vi "SweepCtrlStepCal_DP_ver1.0.vi"(0 "Run Cluster":T1 {"Main Sweep" items=["Time", "DC Current", "Delta Current", "Pulse Delta Current", "Sine Current", "Lock-in Vosc"]; "Magnet Control (IPS 120-10)"."Action" items=["Hold", "To Set point", "To Zero", "Clamp"]; "Keithley 6221 :"."Sweep Mode" items=["Linear", "Log", "Exp", "Inverse", "Manual"]}) -> (1 "Stay duration pts":dbl[](array[numeric]), 2 "2D Array of DC Source or Lock-In Ctrl Run Cluster":cluster{"GPIB ADR":u16, "DC St. Pt.":dbl}[][](array[cluster]))   [LabVIEW 2011]
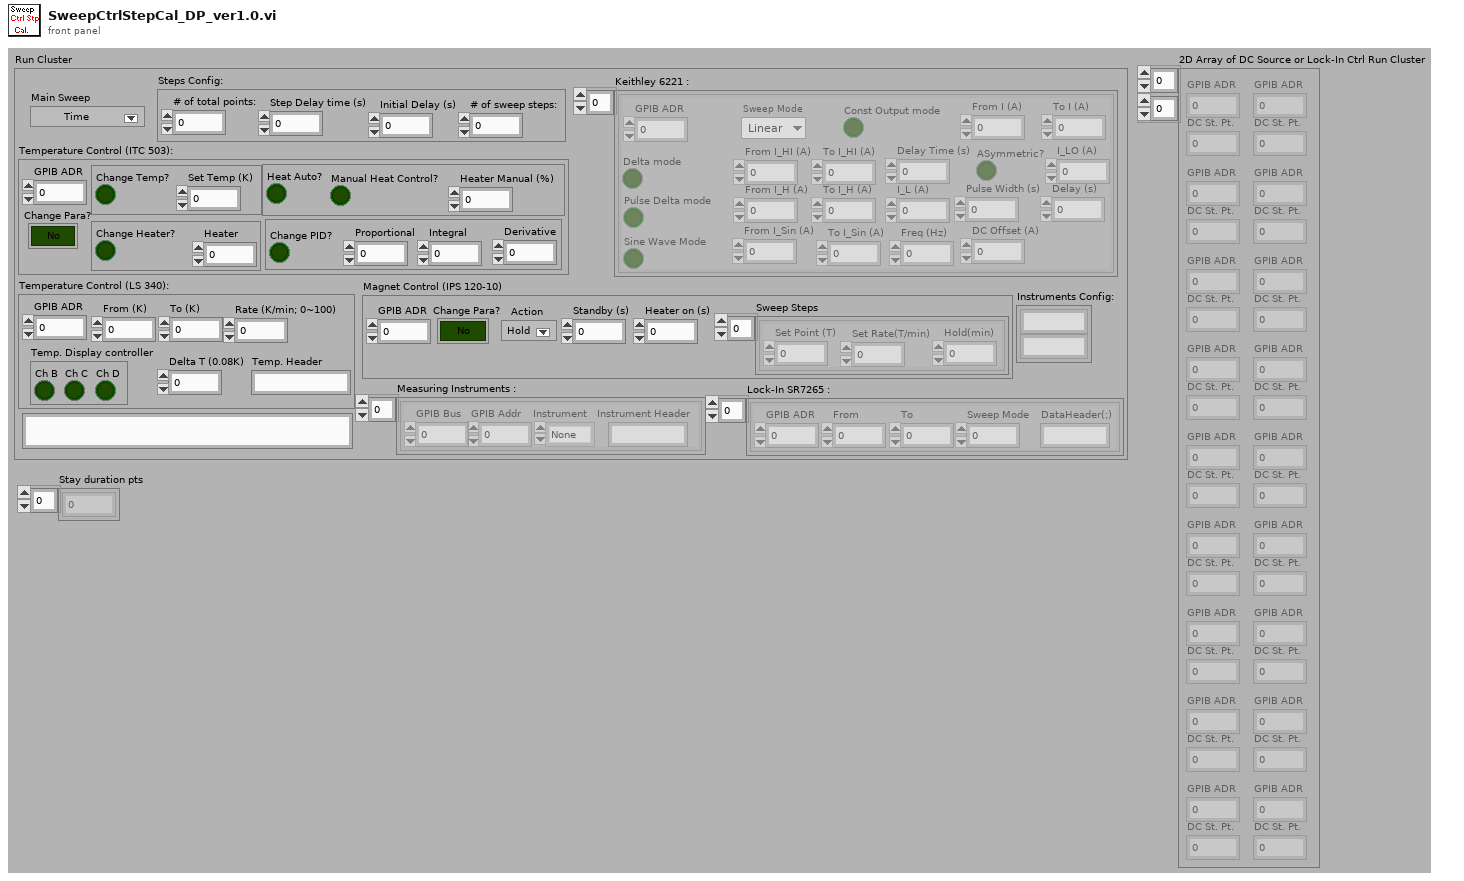
[diagram p1: front panel]
types:
  T1 = cluster{"Main Sweep":u8, "Steps Config:":cluster{"# of total points:":u32, "Step Delay time (s)":dbl, "Initial Delay (s)":dbl, "# of sweep steps:":u32}, "Temperature Control (ITC 503):":cluster{"GPIB ADR":u16, "Change Heater?":cluster{"Change Heater?":bool, "Heater":u8}, "Change Temp?":cluster{"Change Temp?":bool, "Set Temp (K)":dbl}, "Cluster":cluster{"Heat Auto?":bool, "Manual Heat Control?":bool, "Heater Manual (%)":dbl}, "Change PID?":cluster{"Change PID?":bool, "Proportional":dbl, "Integral":dbl, "Derivative":dbl}, "Change Para?":bool}, "Temperature Control (LS 340):":cluster{"GPIB ADR":u16, "From (K)":dbl, "To (K)":dbl, "Rate (K/min; 0~100)":dbl, "Delta T (0.08K)":dbl, "Temp. Header":string, "Temp. Display controller":cluster{"Ch B":bool, "Ch C":bool, "Ch D":bool}}, "Magnet Control (IPS 120-10)":cluster{"Action":u16, "Standby (s)":dbl, "Heater on (s)":dbl, "Sweep Steps ":cluster{"Set Point (T)":dbl, "Set Rate(T/min)":dbl, "Hold(min)":dbl}[], "GPIB ADR":u16, "Change Para?":bool}, "Keithley 6221 :":cluster{"Delta mode":bool, "Const Output mode":bool, "Pulse Delta mode":bool, "Sine Wave Mode":bool, "From I_HI (A)":dbl, "From I (A)":dbl, "I_LO (A)":dbl, "From I_H (A)":dbl, "I_L (A)":dbl, "Freq (Hz)":dbl, "From I_Sin (A)":dbl, "DC Offset (A)":dbl, "Delay Time (s)":dbl, "Pulse Width (s)":dbl, "Delay (s)":dbl, "To I (A)":dbl, "ASymmetric?":bool, "To I_HI (A)":dbl, "To I_H (A)":dbl, "To I_Sin (A)":dbl, "GPIB ADR":u16, "Sweep Mode":u8}[], "Measuring Instruments : ":cluster{"GPIB Bus":dbl, "GPIB Addr":dbl, "Instrument":enum16{"None", "HP34401DMM", "Lockin 7265", "HP3456/7A", "HP3478A", "HP3325FG"}, "Instrument Header":string}[], "Lock-In SR7265 :":cluster{"GPIB ADR":u16, "From":dbl, "To":dbl, "DataHeader(;)":string, "Sweep Mode":u8}[], "Deascription of \nthis measurement":string, "Instruments Config:":string[][]}
  T2 = cluster{"# of total points:":u32, "Step Delay time (s)":dbl, "Initial Delay (s)":dbl, "# of sweep steps:":u32}
  T3 = cluster{"GPIB ADR":u16, "From":dbl, "To":dbl, "DataHeader(;)":string, "Sweep Mode":u8}[]
  T4 = cluster{"Delta mode":bool, "Const Output mode":bool, "Pulse Delta mode":bool, "Sine Wave Mode":bool, "From I_HI (A)":dbl, "From I (A)":dbl, "I_LO (A)":dbl, "From I_H (A)":dbl, "I_L (A)":dbl, "Freq (Hz)":dbl, "From I_Sin (A)":dbl, "DC Offset (A)":dbl, "Delay Time (s)":dbl, "Pulse Width (s)":dbl, "Delay (s)":dbl, "To I (A)":dbl, "ASymmetric?":bool, "To I_HI (A)":dbl, "To I_H (A)":dbl, "To I_Sin (A)":dbl, "GPIB ADR":u16, "Sweep Mode":u8}[]
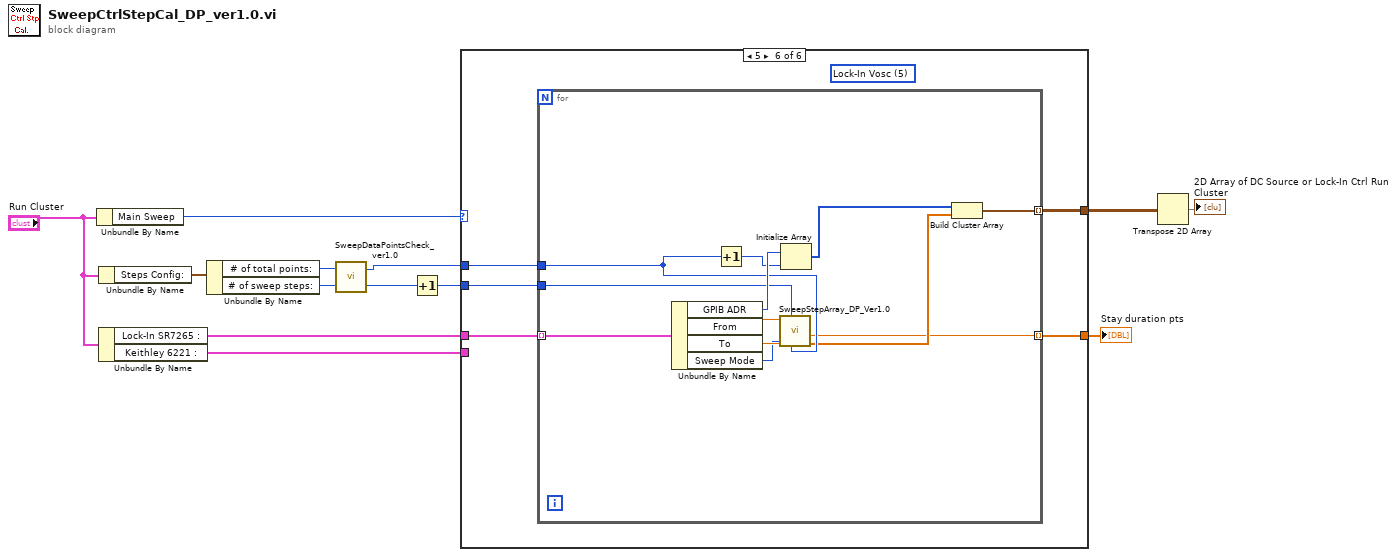
[diagram p0: block diagram]
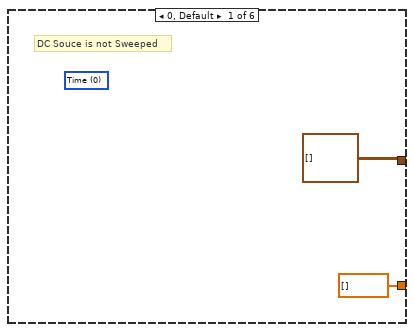
[diagram p2: hidden frame]
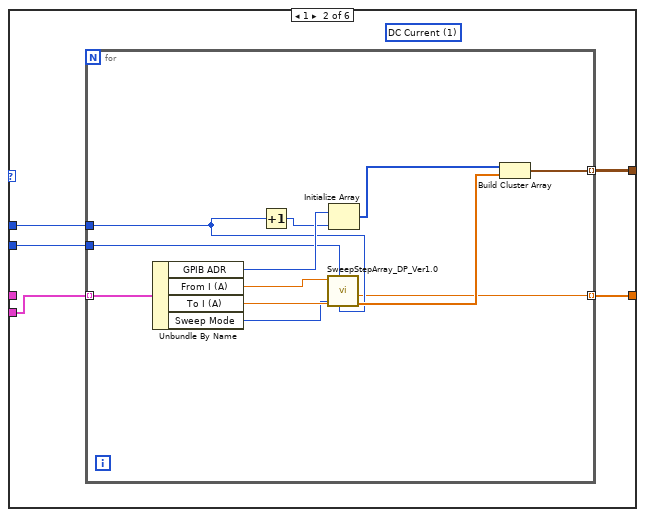
[diagram p3: hidden frame]
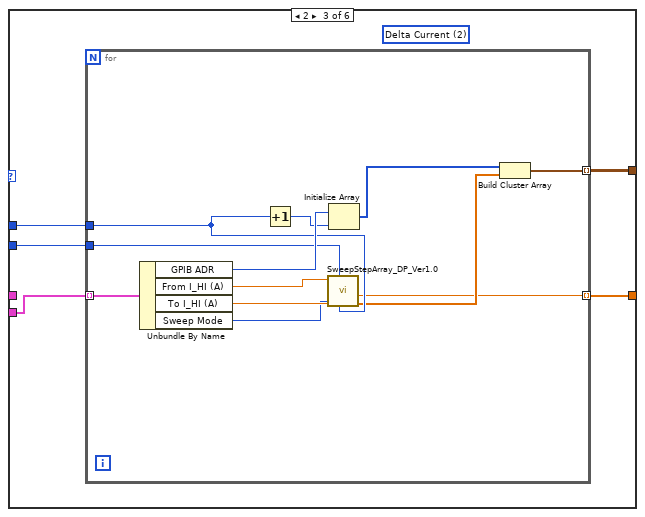
[diagram p4: hidden frame]
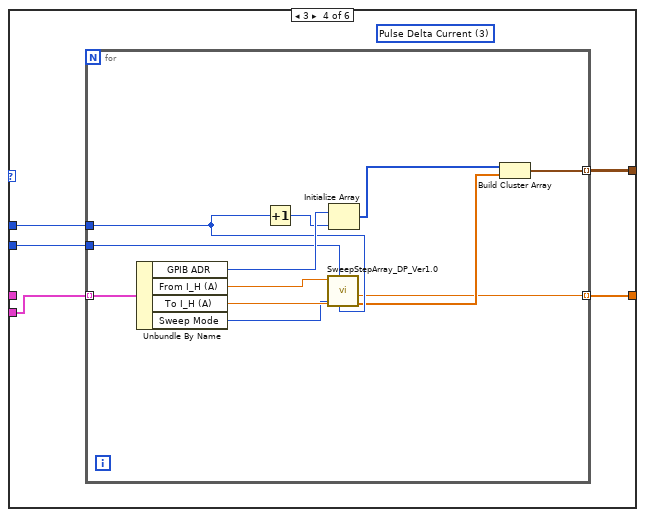
[diagram p5: hidden frame]
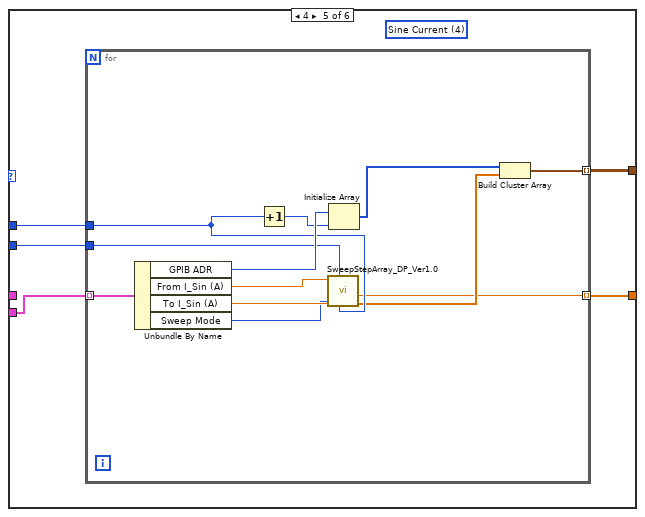
[diagram p6: hidden frame]
diagram:
  n1 = Unbundle By Name("Run Cluster") -> ("Main Sweep"=w11:u8)
  n2 = Unbundle By Name("Run Cluster") -> ("Steps Config:"=w9:T2)
  n3 = Unbundle By Name("Run Cluster") -> ("Lock-In SR7265 :"=w12:T3, "Keithley 6221 :"=w8:T4)
  n4 = Unbundle By Name(w9) -> ("# of total points:"=w7:u32, "# of sweep steps:"=w6:u32)
  n5 = call "SweepDataPointsCheck_ver1.0.vi"("Input # of sweep steps:"=w6, "Input # of total points:"=w7) -> ("Output # of sweep steps:"=w5:u32, "Output # of total points:"=w3:u32)
  n6 = Increment(x=w5) -> (x+1=w4:u32)
  n7 = case shown="5" w11 {
    tunnel: [cluster{"GPIB ADR":u16, "V Start":dbl}[][] [] ("array of clusters") w20 w37 w54 w71 w88] -> w2
    tunnel: w12 -> [_ _ _ _ _ w87]
    tunnel: w3 -> [_ w19 w36 w53 w70 w86]
    tunnel: w4 -> [_ w18 w35 w52 w69 w85]
    tunnel: w8 -> [_ w17 w34 w51 w68 _]
    tunnel: [dbl[] [] w16 w33 w50 w67 w84] -> w1
    frame 0, Default {
      (unwired) u8 0 items=["Time", "DC Current", "Delta Current", "Pulse Delta Current", "Sine Current", "Lock-In Vosc"] ("Main Sweep")
      # "DC Souce is not Sweeped"
    }
    frame 1 {
      (unwired) u8 1 items=["Time", "DC Current", "Delta Current", "Pulse Delta Current", "Sine Current", "Lock-In Vosc"] ("Main Sweep")
      n8 = for {
        tunnel: w17 -> [w32] mode=indexing
        tunnel: [w22] -> w20 mode=indexing
        tunnel: w19 -> [w24]
        tunnel: w18 -> [w27]
        tunnel: [w21] -> w16 mode=indexing
        n9 = Unbundle By Name(w32) -> ("GPIB ADR"=w28:u16, "From I (A)"=w31:dbl, "To I (A)"=w30:dbl, "Sweep Mode"=w29:u8)
        n10 = Increment(x=w24) -> (x+1=w23:u32)
        n11 = call "SweepStepArray_DP_Ver1.0.vi"("# of total points:"=w24, "# of sweep steps:"=w27, "Sweep Mode"=w29, "Stop"=w30, "Start"=w31) -> ("Array Out"=w26:dbl[], "Stay duration points"=w21:dbl)  [unwired: 2 in, 1 out]
        n12 = Initialize Array(w28, w23) -> (w25:u16[])
        n13 = Build Cluster Array(w25, w26) -> (w22:cluster{"GPIB ADR":u16, "V Start":dbl}[])
      }
    }
    frame 2 {
      (unwired) u8 2 items=["Time", "DC Current", "Delta Current", "Pulse Delta Current", "Sine Current", "Lock-In Vosc"] ("Main Sweep")
      n14 = for {
        tunnel: w34 -> [w49] mode=indexing
        tunnel: [w40] -> w37 mode=indexing
        tunnel: w36 -> [w44]
        tunnel: w35 -> [w43]
        tunnel: [w38] -> w33 mode=indexing
        n15 = Unbundle By Name(w49) -> ("GPIB ADR"=w45:u16, "From I_HI (A)"=w48:dbl, "To I_HI (A)"=w47:dbl, "Sweep Mode"=w46:u8)
        n16 = Increment(x=w44) -> (x+1=w39:u32)
        n17 = call "SweepStepArray_DP_Ver1.0.vi"("# of total points:"=w44, "# of sweep steps:"=w43, "Sweep Mode"=w46, "Stop"=w47, "Start"=w48) -> ("Array Out"=w42:dbl[], "Stay duration points"=w38:dbl)  [unwired: 2 in, 1 out]
        n18 = Initialize Array(w45, w39) -> (w41:u16[])
        n19 = Build Cluster Array(w41, w42) -> (w40:cluster{"GPIB ADR":u16, "V Start":dbl}[])
      }
    }
    frame 3 {
      (unwired) u8 3 items=["Time", "DC Current", "Delta Current", "Pulse Delta Current", "Sine Current", "Lock-In Vosc"] ("Main Sweep")
      n20 = for {
        tunnel: w51 -> [w66] mode=indexing
        tunnel: [w57] -> w54 mode=indexing
        tunnel: w53 -> [w61]
        tunnel: w52 -> [w60]
        tunnel: [w55] -> w50 mode=indexing
        n21 = Unbundle By Name(w66) -> ("GPIB ADR"=w62:u16, "From I_H (A)"=w65:dbl, "To I_H (A)"=w64:dbl, "Sweep Mode"=w63:u8)
        n22 = Increment(x=w61) -> (x+1=w56:u32)
        n23 = call "SweepStepArray_DP_Ver1.0.vi"("# of total points:"=w61, "# of sweep steps:"=w60, "Sweep Mode"=w63, "Stop"=w64, "Start"=w65) -> ("Array Out"=w59:dbl[], "Stay duration points"=w55:dbl)  [unwired: 2 in, 1 out]
        n24 = Initialize Array(w62, w56) -> (w58:u16[])
        n25 = Build Cluster Array(w58, w59) -> (w57:cluster{"GPIB ADR":u16, "V Start":dbl}[])
      }
    }
    frame 4 {
      (unwired) u8 4 items=["Time", "DC Current", "Delta Current", "Pulse Delta Current", "Sine Current", "Lock-In Vosc"] ("Main Sweep")
      n26 = for {
        tunnel: w68 -> [w83] mode=indexing
        tunnel: [w74] -> w71 mode=indexing
        tunnel: w70 -> [w78]
        tunnel: w69 -> [w77]
        tunnel: [w72] -> w67 mode=indexing
        n27 = Unbundle By Name(w83) -> ("GPIB ADR"=w79:u16, "From I_Sin (A)"=w82:dbl, "To I_Sin (A)"=w81:dbl, "Sweep Mode"=w80:u8)
        n28 = Increment(x=w78) -> (x+1=w73:u32)
        n29 = call "SweepStepArray_DP_Ver1.0.vi"("# of total points:"=w78, "# of sweep steps:"=w77, "Sweep Mode"=w80, "Stop"=w81, "Start"=w82) -> ("Array Out"=w76:dbl[], "Stay duration points"=w72:dbl)  [unwired: 2 in, 1 out]
        n30 = Initialize Array(w79, w73) -> (w75:u16[])
        n31 = Build Cluster Array(w75, w76) -> (w74:cluster{"GPIB ADR":u16, "V Start":dbl}[])
      }
    }
    frame 5 {
      (unwired) u8 5 items=["Time", "DC Current", "Delta Current", "Pulse Delta Current", "Sine Current", "Lock-In Vosc"] ("Main Sweep")
      n32 = for {
        tunnel: w87 -> [w100] mode=indexing
        tunnel: [w91] -> w88 mode=indexing
        tunnel: w86 -> [w95]
        tunnel: w85 -> [w94]
        tunnel: [w89] -> w84 mode=indexing
        n33 = Unbundle By Name(w100) -> ("GPIB ADR"=w96:u16, "From"=w99:dbl, "To"=w98:dbl, "Sweep Mode"=w97:u8)
        n34 = Increment(x=w95) -> (x+1=w90:u32)
        n35 = call "SweepStepArray_DP_Ver1.0.vi"("# of total points:"=w95, "# of sweep steps:"=w94, "Sweep Mode"=w97, "Stop"=w98, "Start"=w99) -> ("Array Out"=w93:dbl[], "Stay duration points"=w89:dbl)  [unwired: 2 in, 1 out]
        n36 = Initialize Array(w96, w90) -> (w92:u16[])
        n37 = Build Cluster Array(w92, w93) -> (w91:cluster{"GPIB ADR":u16, "V Start":dbl}[])
      }
    }
  }
  "Stay duration pts" <- w1
  n38 = Transpose 2D Array(2D array=w2) -> (transposed array=→"2D Array of DC Source or Lock-In Ctrl Run Cluster":cluster{"GPIB ADR":u16, "V Start":dbl}[][])
